vi "CRYAPI REMOVE.vi"(6 "sData":string, 8 "nData":i32, 9 "tFrame":T3, 10 "List_ID":i32[](array[numeric]), 11 "sAction":string) -> (0 "nData_Out":i32, 1 "tSpliter_Out":T1, 2 "tFrame_Out":T3, 3 "List_ID_Out":i32[](array[numeric]))   [LabVIEW 2013]
uses:
  <vilib>/Utility/miscctls.llb/LVRectTypeDef.ctl
  CRYMain Sub Window Global.vi
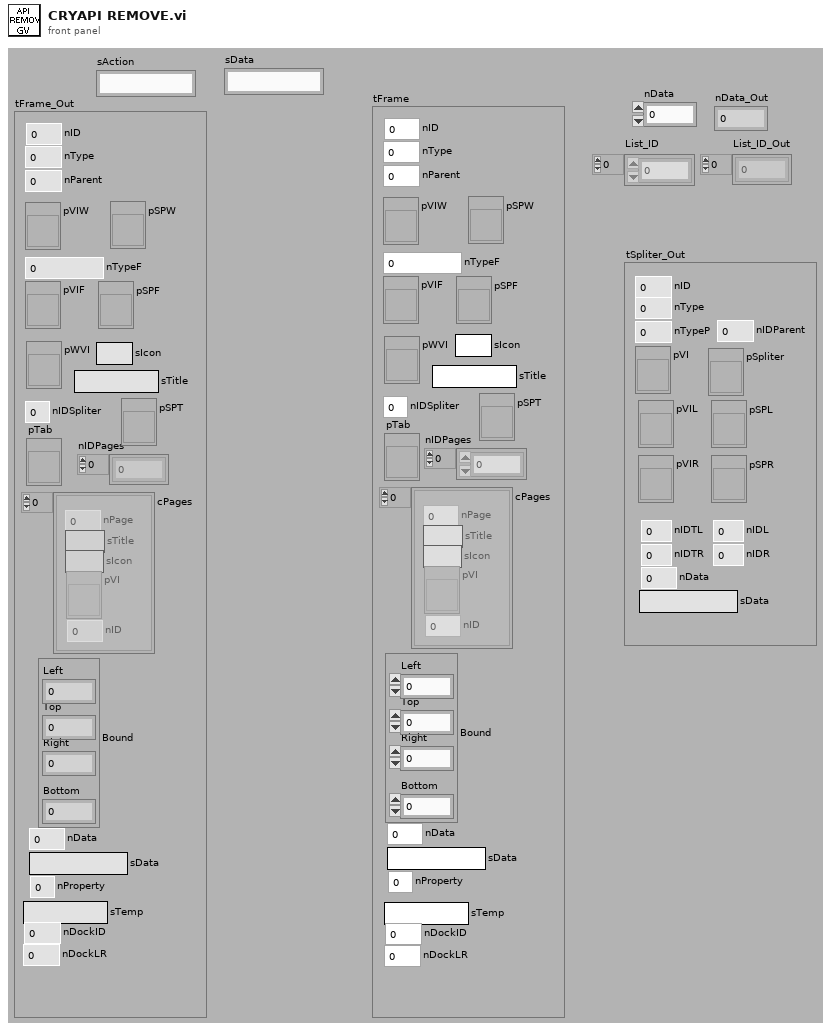
[diagram p1: front panel]
types:
  T1 = cluster{"nType":i32, "nTypeP":i32, "pVI":refnum<vi>, "pSpliter":refnum<vi>, "pSPL":refnum<vi>, "pVIL":refnum<vi>, "pSPR":refnum<vi>, "pVIR":refnum<vi>, "nIDTL":i32, "nIDL":i32, "nIDTR":i32, "nIDR":i32, "nID":i32, "nIDParent":i32, "nData":i32, "sData":string}
  T2 = typedef "LVRectTypeDef.ctl" = cluster{"Left":i16, "Top":i16, "Right":i16, "Bottom":i16}
  T3 = cluster{"nType":i32, "nParent":i32, "pVIW":refnum<vi>, "pSPW":refnum<vi>, "nTypeF":i32, "pVIF":refnum<vi>, "pSPF":refnum<vi>, "nIDSpliter":i32, "nProperty":i32, "Bound":T2, "nID":i32, "nData":i32, "sData":string, "pWVI":refnum<vi>, "sTitle":string, "cPages":cluster{"nPage":i32, "sTitle":string, "sIcon":string, "pVI":refnum<vi>, "nID":i32}[], "pTab":refnum<vi>, "nIDPages":i32[], "pSPT":refnum<vi>, "sTemp":string, "nDockID":i32, "nDockLR":i32, "sIcon":string}
  T4 = enum32{"Invalid", "Standard", "Closed", "Hidden", "Minimized", "Maximized"}
  T5 = cluster{"nPage":i32, "sTitle":string, "sIcon":string, "pVI":refnum<vi>, "nID":i32}[]
  T6 = cluster{"pSP":refnum<vi>, "pVI":refnum<vi>, "nIDT":i32, "nID":i32, "nLR":i32}
  T7 = cluster{"nID":i32[], "Frame":cluster{"nType":i32, "nParent":i32, "pVIW":refnum<vi>, "pSPW":refnum<vi>, "nTypeF":i32, "pVIF":refnum<vi>, "pSPF":refnum<vi>, "nIDSpliter":i32, "nProperty":i32, "Bound":T2, "nID":i32, "nData":i32, "sData":string, "pWVI":refnum<vi>, "sTitle":string, "cPages":cluster{"nPage":i32, "sTitle":string, "sIcon":string, "pVI":refnum<vi>, "nID":i32}[], "pTab":refnum<vi>, "nIDPages":i32[], "pSPT":refnum<vi>, "sTemp":string, "nDockID":i32, "nDockLR":i32, "sIcon":string}[]}
  T8 = cluster{"nType":i32, "nParent":i32, "pVIW":refnum<vi>, "pSPW":refnum<vi>, "nTypeF":i32, "pVIF":refnum<vi>, "pSPF":refnum<vi>, "nIDSpliter":i32, "nProperty":i32, "Bound":T2, "nID":i32, "nData":i32, "sData":string, "pWVI":refnum<vi>, "sTitle":string, "cPages":cluster{"nPage":i32, "sTitle":string, "sIcon":string, "pVI":refnum<vi>, "nID":i32}[], "pTab":refnum<vi>, "nIDPages":i32[], "pSPT":refnum<vi>, "sTemp":string, "nDockID":i32, "nDockLR":i32, "sIcon":string}[]
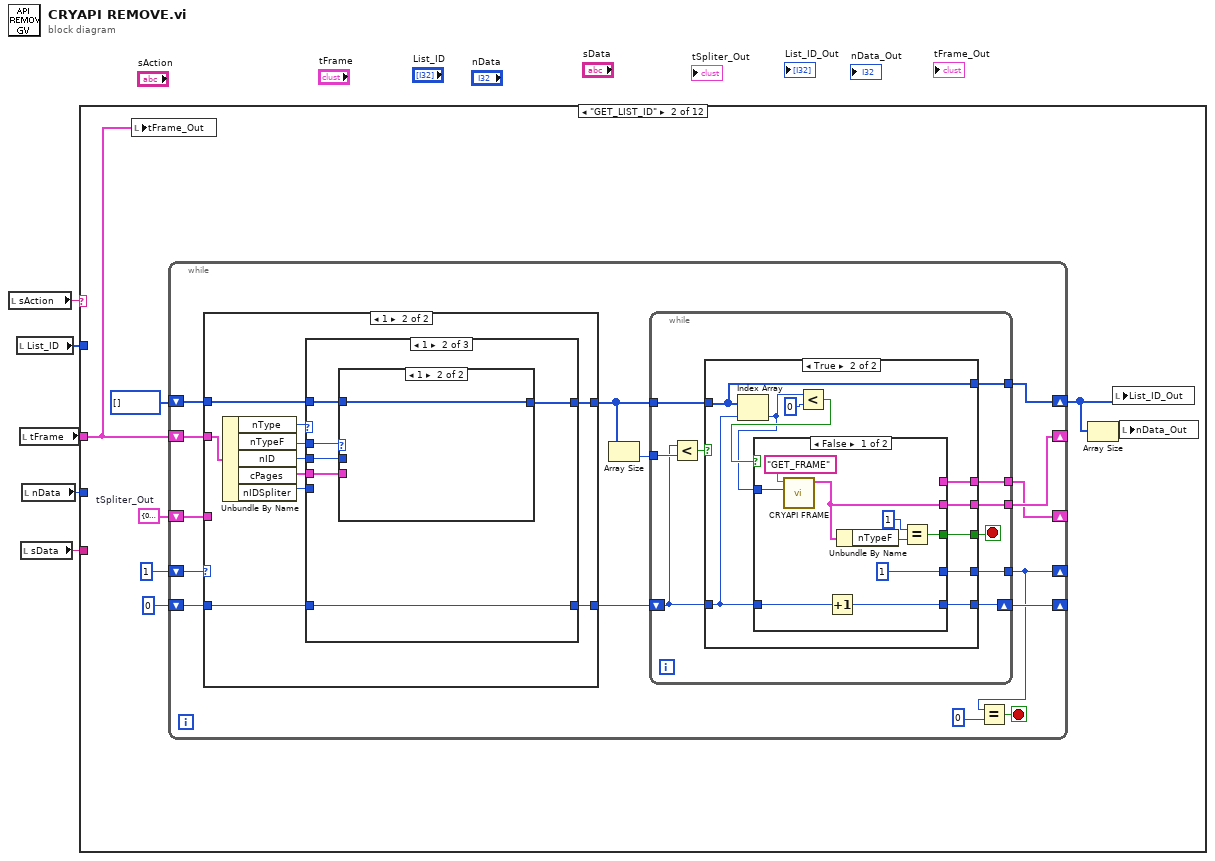
[diagram p0: block diagram]
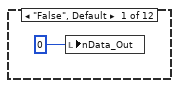
[diagram p2: hidden frame]
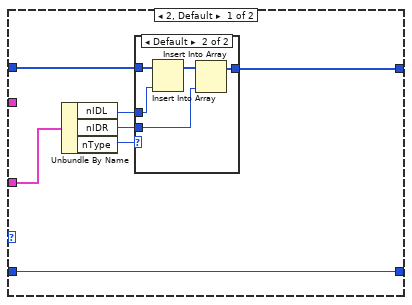
[diagram p3: hidden frame]
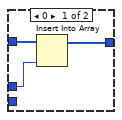
[diagram p4: hidden frame]
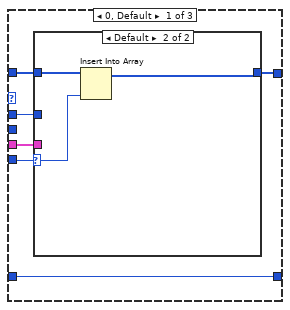
[diagram p5: hidden frame]
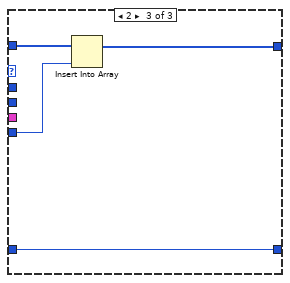
[diagram p8: hidden frame]
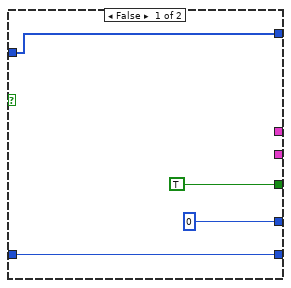
[diagram p9: hidden frame]
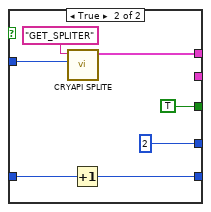
[diagram p10: hidden frame]
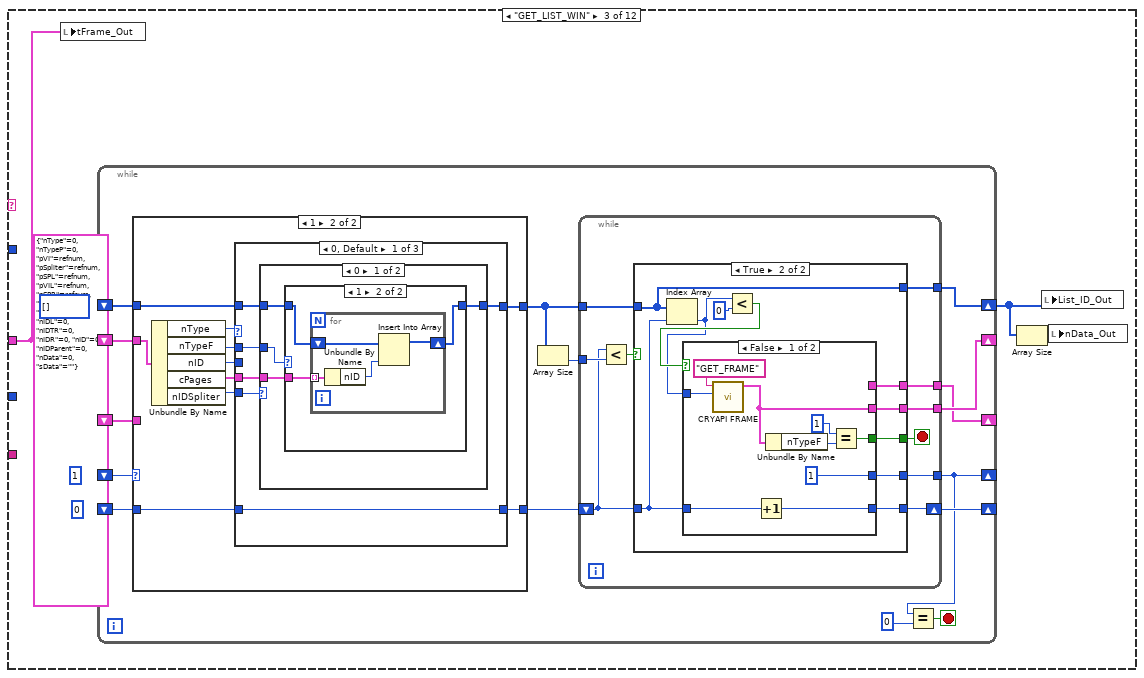
[diagram p11: hidden frame]
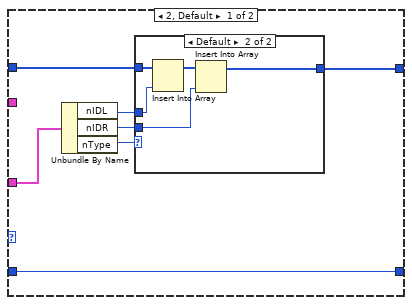
[diagram p12: hidden frame]
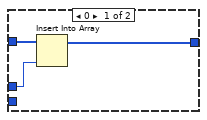
[diagram p13: hidden frame]
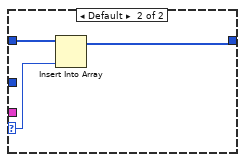
[diagram p15: hidden frame]
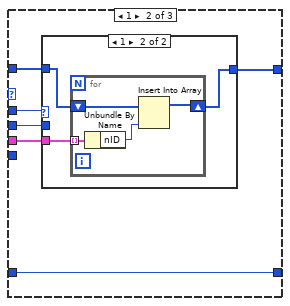
[diagram p16: hidden frame]
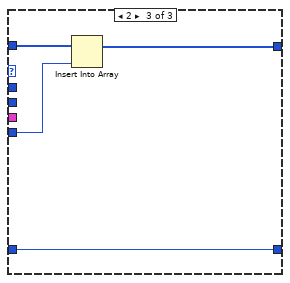
[diagram p18: hidden frame]
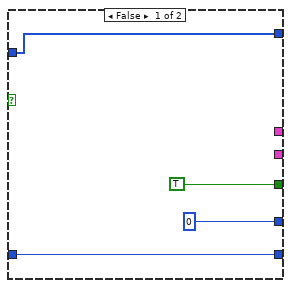
[diagram p19: hidden frame]
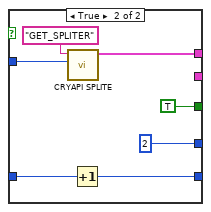
[diagram p20: hidden frame]
diagram:
  n1 = local read "sAction"() -> (w5:string)
  n2 = local read "List_ID"() -> (w3:i32[])
  n3 = local read "tFrame"() -> (w4:T3)
  n4 = local read "sData"() -> (w1:string)
  n5 = local read "nData"() -> (w2:i32)
  n6 = case shown="\"GET_LIST_ID\"" w5 {
    selector: w5 -> [_ _ _ _ w253 w299 _ _ w406 w455 w478 _]
    tunnel: w4 -> [_ w7 w116 w246 _ _ w362 _ _ _ _ _]
    tunnel: w3 -> [_ _ _ _ w255 w298 w364 w374 _ _ _ w518]
    tunnel: w2 -> [_ _ _ _ _ _ _ w379 _ _ _ w517]
    tunnel: w1 -> [_ _ _ _ _ _ _ _ _ _ _ _]
    frame "False", Default {
      n7 = local write "nData_Out"(0 ("nData_Out")) -> ()
    }
    frame "GET_LIST_ID" {
      w10 = T1 {"nType"=0, "nTypeP"=0, "pVI"=refnum, "pSpliter"=refnum, "pSPL"=refnum, "pVIL"=refnum, "pSPR"=refnum, "pVIR"=refnum, "nIDTL"=0, "nIDL"=0, "nIDTR"=0, "nIDR"=0, "nID"=0, "nIDParent"=0, "nData"=0, "sData"=""}  # tSpliter_Out
      n8 = local write "tFrame_Out"(w7) -> ()
      n9 = while {
        shift-right: [w22] -> _
        shift-left: w7 -> [w28]
        shift-right: [w14] -> w8
        shift-left: i32[] [] ("List_nID") -> [w27]
        shift-right: [w21] -> _
        shift-left: 0 -> [w26]
        shift-right: [w18] -> _
        shift-left: 1 -> [w16]
        shift-right: [w17] -> _
        shift-left: w10 -> [w15]
        stop <- w19 stop-if-true
        n10 = case shown="1" w16 {
          tunnel: w28 -> [_ w53]
          tunnel: w27 -> [w32 w49]
          tunnel: w26 -> [w30 w46]
          tunnel: [w31 w45] -> w25
          tunnel: [w30 w44] -> w23
          tunnel: w15 -> [w33 _]
          frame 2, Default {
            n11 = Unbundle By Name(w33) -> ("nIDL"=w34:i32, "nIDR"=w35:i32, "nType"=w29:i32)
            n12 = case shown="Default" w29 {
              tunnel: w35 -> [_ w43]
              tunnel: w34 -> [w38 w41]
              tunnel: w32 -> [w37 w40]
              tunnel: [w36 w39] -> w31
              frame 0 {
                n13 = Insert Into Array(array=w37, new element=w38) -> (w36:i32[])  [unwired: 1 in]
              }
              frame Default {
                n14 = Insert Into Array(array=w40, new element=w41) -> (w42:i32[])  [unwired: 1 in]
                n15 = Insert Into Array(array=w42, new element=w43) -> (w39:i32[])  [unwired: 1 in]
              }
            }
          }
          frame 1 {
            n16 = Unbundle By Name(w53) -> ("nType"=w52:i32, "nTypeF"=w51:i32, "nID"=w50:i32, "cPages"=w48:T5, "nIDSpliter"=w47:i32)
            n17 = case shown="1" w52 {
              tunnel: w51 -> [w57 w69 _]
              tunnel: w50 -> [_ w68 _]
              tunnel: w49 -> [w59 w67 w75]
              tunnel: [w56 w66 w74] -> w45
              tunnel: w48 -> [w55 w65 _]
              tunnel: w47 -> [w58 _ w72]
              tunnel: w46 -> [w54 w64 w73]
              tunnel: [w54 w64 w73] -> w44
              frame 0, Default {
                n18 = case shown="Default" w58 {
                  selector: w58 -> [_ w62]
                  tunnel: w59 -> [w60 w63]
                  tunnel: w57 -> [_ _]
                  tunnel: [w60 w61] -> w56
                  tunnel: w55 -> [_ _]
                  frame 0 {
                  }
                  frame Default {
                    n19 = Insert Into Array(array=w63, new element=w62) -> (w61:i32[])  [unwired: 1 in]
                  }
                }
              }
              frame 1 {
                n20 = case shown="1" w69 {
                  tunnel: w68 -> [_ _]
                  tunnel: w67 -> [w70 w71]
                  tunnel: [w70 w71] -> w66
                  tunnel: w65 -> [_ _]
                  frame 0, Default {
                  }
                  frame 1 {
                  }
                }
              }
              frame 2 {
                n21 = Insert Into Array(array=w75, new element=w72) -> (w74:i32[])  [unwired: 1 in]
              }
            }
          }
        }
        n22 = Array Size(array=w25) -> (size(s)=w24:i32)
        n23 = while {
          tunnel: w25 -> [w83]
          tunnel: w24 -> [w84]
          shift-right: [w78] -> w21
          shift-left: w23 -> [w82]
          tunnel: [w81] -> w17
          tunnel: [w80] -> w22
          tunnel: [w79] -> w18
          tunnel: [w76] -> w14
          stop <- w77 stop-if-true
          n24 = Less?(x=w82, y=w84) -> (x < y?=w85:bool)
          n25 = case shown="True" w85 {
            tunnel: w83 -> [w86 w90]
            tunnel: w82 -> [w88 w93]
            tunnel: [_ w96] -> w81
            tunnel: [_ w95] -> w80
            tunnel: [0 w94] -> w79
            tunnel: [w88 w92] -> w78
            tunnel: [TRUE w91] -> w77
            tunnel: [w86 w90] -> w76
            frame False {
            }
            frame True {
              n26 = Index Array(array=w90, index=w93) -> (element=w97:i32)
              n27 = Less?(x=w97, y=0) -> (x < y?=w98:bool)
              n28 = case shown="False" w98 {
                tunnel: w97 -> [w107 w114]
                tunnel: [_ w113] -> w96
                tunnel: [w103 _] -> w95
                tunnel: [1 2] -> w94
                tunnel: w93 -> [w105 w111]
                tunnel: [w104 w110] -> w92
                tunnel: [w100 TRUE] -> w91
                frame False {
                  n29 = call "CRYAPI FRAME.vi"("nData"=w107, "sAction"="GET_FRAME") -> ("tFrame_Out"=w103:T3)  [unwired: 4 in, 5 out]
                  n30 = Increment(x=w105) -> (x+1=w104:i32)
                  n31 = Unbundle By Name(w103) -> ("nTypeF"=w101:i32)
                  n32 = Equal?(x=1 ("y"), y=w101) -> (x = y?=w100:bool)
                }
                frame True {
                  n33 = call "CRYAPI SPLITE.vi"("nData"=w114, "sAction"="GET_SPLITER") -> ("tSpliter_Out"=w113:T1)  [unwired: 4 in, 5 out]
                  n34 = Increment(x=w111) -> (x+1=w110:i32)
                }
              }
            }
          }
        }
        n35 = Equal?(x=w18, y=0 ("x")) -> (x = y?=w19:bool)
      }
      n36 = Array Size(array=w8) -> (size(s)=w9:i32)
      n37 = local write "List_ID_Out"(w8) -> ()
      n38 = local write "nData_Out"(w9) -> ()
    }
    frame "GET_LIST_WIN" {
      n39 = local write "tFrame_Out"(w116) -> ()
      n40 = while {
        shift-right: [w131] -> _
        shift-left: w116 -> [w137]
        shift-right: [w123] -> w117
        shift-left: i32[] [] ("List_nID") -> [w136]
        shift-right: [w130] -> _
        shift-left: 0 -> [w135]
        shift-right: [w127] -> _
        shift-left: 1 -> [w125]
        shift-right: [w126] -> _
        shift-left: T1 {"nType"=0, "nTypeP"=0, "pVI"=refnum, "pSpliter"=refnum, "pSPL"=refnum, "pVIL"=refnum, "pSPR"=refnum, "pVIR"=refnum, "nIDTL"=0, "nIDL"=0, "nIDTR"=0, "nIDR"=0, "nID"=0, "nIDParent"=0, "nData"=0, "sData"=""} ("tSpliter_Out") -> [w124]
        stop <- w128 stop-if-true
        n41 = case shown="1" w125 {
          tunnel: w137 -> [_ w162]
          tunnel: w136 -> [w141 w158]
          tunnel: w135 -> [w139 w155]
          tunnel: [w140 w154] -> w134
          tunnel: [w139 w153] -> w132
          tunnel: w124 -> [w142 _]
          frame 2, Default {
            n42 = Unbundle By Name(w142) -> ("nIDL"=w143:i32, "nIDR"=w144:i32, "nType"=w138:i32)
            n43 = case shown="Default" w138 {
              tunnel: w144 -> [_ w152]
              tunnel: w143 -> [w147 w150]
              tunnel: w141 -> [w146 w149]
              tunnel: [w145 w148] -> w140
              frame 0 {
                n44 = Insert Into Array(array=w146, new element=w147) -> (w145:i32[])  [unwired: 1 in]
              }
              frame Default {
                n45 = Insert Into Array(array=w149, new element=w150) -> (w151:i32[])  [unwired: 1 in]
                n46 = Insert Into Array(array=w151, new element=w152) -> (w148:i32[])  [unwired: 1 in]
              }
            }
          }
          frame 1 {
            n47 = Unbundle By Name(w162) -> ("nType"=w161:i32, "nTypeF"=w160:i32, "nID"=w159:i32, "cPages"=w157:T5, "nIDSpliter"=w156:i32)
            n48 = case shown="0, Default" w161 {
              tunnel: w160 -> [w166 w189 _]
              tunnel: w159 -> [_ w188 _]
              tunnel: w158 -> [w168 w187 w201]
              tunnel: [w165 w186 w200] -> w154
              tunnel: w157 -> [w164 w185 _]
              tunnel: w156 -> [w167 _ w198]
              tunnel: w155 -> [w163 w184 w199]
              tunnel: [w163 w184 w199] -> w153
              frame 0, Default {
                n49 = case shown="0" w167 {
                  selector: w167 -> [_ w181]
                  tunnel: w168 -> [w171 w183]
                  tunnel: w166 -> [w169 _]
                  tunnel: [w170 w182] -> w165
                  tunnel: w164 -> [w172 _]
                  frame 0 {
                    n50 = case shown="1" w169 {
                      tunnel: w172 -> [_ w176]
                      tunnel: w171 -> [w173 w175]
                      tunnel: [w173 w174] -> w170
                      frame 0, Default {
                      }
                      frame 1 {
                        n51 = for {
                          tunnel: w176 -> [w180] mode=indexing
                          shift-right: [w177] -> w174
                          shift-left: w175 -> [w178]
                          n52 = Unbundle By Name(w180) -> ("nID"=w179:i32)
                          n53 = Insert Into Array(array=w178, new element=w179) -> (w177:i32[])  [unwired: 1 in]
                        }
                      }
                    }
                  }
                  frame Default {
                    n54 = Insert Into Array(array=w183, new element=w181) -> (w182:i32[])  [unwired: 1 in]
                  }
                }
              }
              frame 1 {
                n55 = case shown="1" w189 {
                  tunnel: w188 -> [_ _]
                  tunnel: w187 -> [w190 w192]
                  tunnel: [w190 w191] -> w186
                  tunnel: w185 -> [_ w193]
                  frame 0, Default {
                  }
                  frame 1 {
                    n56 = for {
                      tunnel: w193 -> [w197] mode=indexing
                      shift-right: [w194] -> w191
                      shift-left: w192 -> [w195]
                      n57 = Unbundle By Name(w197) -> ("nID"=w196:i32)
                      n58 = Insert Into Array(array=w195, new element=w196) -> (w194:i32[])  [unwired: 1 in]
                    }
                  }
                }
              }
              frame 2 {
                n59 = Insert Into Array(array=w201, new element=w198) -> (w200:i32[])  [unwired: 1 in]
              }
            }
          }
        }
        n60 = Array Size(array=w134) -> (size(s)=w133:i32)
        n61 = while {
          tunnel: w134 -> [w209]
          tunnel: w133 -> [w210]
          shift-right: [w204] -> w130
          shift-left: w132 -> [w208]
          tunnel: [w207] -> w126
          tunnel: [w206] -> w131
          tunnel: [w205] -> w127
          tunnel: [w202] -> w123
          stop <- w203 stop-if-true
          n62 = Less?(x=w208, y=w210) -> (x < y?=w211:bool)
          n63 = case shown="True" w211 {
            tunnel: w209 -> [w212 w216]
            tunnel: w208 -> [w214 w219]
            tunnel: [_ w222] -> w207
            tunnel: [_ w221] -> w206
            tunnel: [0 w220] -> w205
            tunnel: [w214 w218] -> w204
            tunnel: [TRUE w217] -> w203
            tunnel: [w212 w216] -> w202
            frame False {
            }
            frame True {
              n64 = Index Array(array=w216, index=w219) -> (element=w223:i32)
              n65 = Less?(x=w223, y=0) -> (x < y?=w224:bool)
              n66 = case shown="False" w224 {
                tunnel: w223 -> [w233 w240]
                tunnel: [_ w239] -> w222
                tunnel: [w229 _] -> w221
                tunnel: [1 2] -> w220
                tunnel: w219 -> [w231 w237]
                tunnel: [w230 w236] -> w218
                tunnel: [w226 TRUE] -> w217
                frame False {
                  n67 = call "CRYAPI FRAME.vi"("nData"=w233, "sAction"="GET_FRAME") -> ("tFrame_Out"=w229:T3)  [unwired: 4 in, 5 out]
                  n68 = Increment(x=w231) -> (x+1=w230:i32)
                  n69 = Unbundle By Name(w229) -> ("nTypeF"=w227:i32)
                  n70 = Equal?(x=1 ("y"), y=w227) -> (x = y?=w226:bool)
                }
                frame True {
                  n71 = call "CRYAPI SPLITE.vi"("nData"=w240, "sAction"="GET_SPLITER") -> ("tSpliter_Out"=w239:T1)  [unwired: 4 in, 5 out]
                  n72 = Increment(x=w237) -> (x+1=w236:i32)
                }
              }
            }
          }
        }
        n73 = Equal?(x=w127, y=0 ("x")) -> (x = y?=w128:bool)
      }
      n74 = Array Size(array=w117) -> (size(s)=w118:i32)
      n75 = local write "List_ID_Out"(w117) -> ()
      n76 = local write "nData_Out"(w118) -> ()
    }
    frame "GET_LIST_PAGES" {
      n77 = Unbundle By Name(w246) -> ("cPages"=w245:T5)
      n78 = for {
        tunnel: w245 -> [w250] mode=indexing
        shift-right: [w247] -> w242
        shift-left: i32[] [] ("List_nID") -> [w249]
        n79 = Unbundle By Name(w250) -> ("nID"=w248:i32)
        n80 = Insert Into Array(array=w249, new element=w248) -> (w247:i32[])  [unwired: 1 in]
      }
      n81 = Array Size(array=w242) -> (size(s)=w243:i32)
      n82 = local write "List_ID_Out"(w242) -> ()
      n83 = local write "nData_Out"(w243) -> ()
    }
    frame "GET_LIST_IDFRAME", "GET_LIST_IDSPLITER", "GET_LIST_IDWIN" {
      n84 = for {
        tunnel: w255 -> [w258] mode=indexing
        shift-right: [w257] -> w251
        shift-left: i32[] [] ("List_ID") -> [w260]
        tunnel: w253 -> [w256]
        n85 = case shown="\"GET_LIST_IDFRAME\"" w256 {
          tunnel: [w261 w264 w279] -> w259
          tunnel: w258 -> [w262 w265 w280]
          frame "GET_LIST_IDSPLITER", Default {
            n86 = Less?(x=w262, y=0) -> (x < y?=w261:bool)
          }
          frame "GET_LIST_IDWIN" {
            n87 = Greater?(x=w265, y=0) -> (0:w266:bool)
            n88 = case shown="True" w266 {
              tunnel: w265 -> [_ w277]
              tunnel: [FALSE w269] -> w264
              frame False {
              }
              frame True {
                n89 = call "CRYAPI FRAME.vi"("nData"=w277, "sAction"="GET_FRAME") -> ("tFrame_Out"=w276:T3)  [unwired: 4 in, 5 out]
                n90 = Unbundle By Name(w276) -> ("nType"=w274:i32, "nTypeF"=w275:i32)
                n91 = Equal?(x=1, y=w274) -> (x = y?=w270:bool)
                n92 = Equal?(x=w275, y=0 ("x")) -> (x = y?=w271:bool)
                n93 = And(x=w270, y=w271) -> (x .and. y?=w269:bool)
              }
            }
          }
          frame "GET_LIST_IDFRAME" {
            n94 = Greater?(x=w280, y=0) -> (0:w281:bool)
            n95 = case shown="True" w281 {
              tunnel: w280 -> [_ w292]
              tunnel: [FALSE w284] -> w279
              frame False {
              }
              frame True {
                n96 = call "CRYAPI FRAME.vi"("nData"=w292, "sAction"="GET_FRAME") -> ("tFrame_Out"=w291:T3)  [unwired: 4 in, 5 out]
                n97 = Unbundle By Name(w291) -> ("nType"=w289:i32, "nTypeF"=w290:i32)
                n98 = Equal?(x=2, y=w289) -> (x = y?=w285:bool)
                n99 = Equal?(x=w290, y=1 ("x")) -> (x = y?=w286:bool)
                n100 = Or(x=w285, y=w286) -> (x .or. y?=w284:bool)
              }
            }
          }
        }
        n101 = case shown="True" w259 {
          tunnel: w260 -> [w294 w297]
          tunnel: w258 -> [_ w296]
          tunnel: [w294 w295] -> w257
          frame False {
          }
          frame True {
            n102 = Insert Into Array(array=w297, new element=w296) -> (w295:i32[])  [unwired: 1 in]
          }
        }
      }
      n103 = Array Size(array=w251) -> (size(s)=w252:i32)
      n104 = local write "List_ID_Out"(w251) -> ()
      n105 = local write "nData_Out"(w252) -> ()
    }
    frame "REMOVE_FRAMES", "REMOVE_FRAME_ONLY", "REMOVE_SPF", "REMOVE_SPLITERS" {
      n106 = local write "List_ID_Out"(w298) -> ()
      n107 = for {
        tunnel: w298 -> [w301] mode=indexing
        tunnel: w299 -> [w300]
        n108 = case shown="\"REMOVE_SPF\"" w300 {
          tunnel: w301 -> [w302 w306 w311 w312]
          frame "REMOVE_FRAMES", Default {
            n109 = call "CRYAPI FRAME LIB.vi"("nData"=w302, "sAction"="REMOVE_FRAME") -> ()  [unwired: 4 in, 6 out]
          }
          frame "REMOVE_FRAME_ONLY" {
            n110 = call "CRYAPI FRAME.vi"("nData"=w306, "sAction"="GET_FRAME") -> ("tFrame_Out"=w304:T3)  [unwired: 4 in, 5 out]
            n111 = call "CRYAPI FRAME.vi"("tFrame"=w304, "sAction"="REMOVE_FRAME") -> ()  [unwired: 4 in, 6 out]
          }
          frame "REMOVE_SPLITERS" {
            n112 = call "CRYAPI SPLITE.vi"("nData"=w311, "sAction"="GET_SPLITER") -> ("tSpliter_Out"=w308:T1)  [unwired: 4 in, 5 out]
            n113 = call "CRYAPI SPLITE.vi"("tSpliter"=w308, "sAction"="REMOVE_SPLITER") -> ()  [unwired: 4 in, 6 out]
          }
          frame "REMOVE_SPF" {
            n114 = Less?(x=w312, y=0) -> (x < y?=w313:bool)
            n115 = case shown="False" w313 {
              tunnel: w312 -> [w319 w335]
              frame False {
                n116 = call "CRYAPI FRAME.vi"("nData"=w319, "sAction"="GET_FRAME") -> ("tFrame_Out"=w318:T3)  [unwired: 4 in, 5 out]
                n117 = Unbundle By Name(w318) -> ("nType"=w317:i32)
                n118 = Not Equal?(x=w317, y=1) -> (x != y?=w315:bool)
                n119 = case shown="True" w315 {
                  tunnel: w318 -> [_ w321]
                  frame False {
                  }
                  frame True {
                    n120 = Bundle By Name(cluster=w321, "nIDSpliter"=0) -> (w322:T3)
                    n121 = Unbundle By Name(w321) -> ("pSPF"=w325:refnum<vi>)
                    n122 = invoke class="SubPnl" method="Remove VI"(reference=w325) -> ()  [unwired: 2 in, 3 out]
                    n123 = call "CRYAPI FRAME.vi"("tFrame"=w322, "sAction"="REPLACE_FRAME") -> ()  [unwired: 4 in, 6 out]
                  }
                }
              }
              frame True {
                n124 = call "CRYAPI SPLITE.vi"("nData"=w335, "sAction"="GET_SPLITER") -> ("tSpliter_Out"=w326:T1)  [unwired: 4 in, 5 out]
                n125 = Unbundle By Name(w326) -> ("pSPL"=w332:refnum<vi>, "pSPR"=w331:refnum<vi>, "nType"=w333:i32, "nTypeP"=w330:i32, "nIDParent"=w328:i32)
                n126 = case shown="Default" w333 {
                  tunnel: w332 -> [w355 w359]
                  tunnel: w331 -> [_ w358]
                  tunnel: w330 -> [w354 w357]
                  tunnel: [w354 w357] -> w329
                  tunnel: w328 -> [w353 w356]
                  tunnel: [w353 w356] -> w327
                  frame 0 {
                    n127 = invoke class="SubPnl" method="Remove VI"(reference=w355) -> ()  [unwired: 2 in, 3 out]
                  }
                  frame Default {
                    n128 = invoke class="SubPnl" method="Remove VI"(reference=w358) -> ()  [unwired: 2 in, 3 out]
                    n129 = invoke class="SubPnl" method="Remove VI"(reference=w359) -> ()  [unwired: 2 in, 3 out]
                  }
                }
                n130 = case shown="0, Default" w329 {
                  tunnel: w327 -> [w341 w350]
                  tunnel: w326 -> [_ w348]
                  frame 0, Default {
                    n131 = call "CRYAPI FRAME.vi"("nData"=w341, "sAction"="GET_FRAME") -> ("tFrame_Out"=w337:T3)  [unwired: 4 in, 5 out]
                    n132 = Unbundle By Name(w337) -> ("pSPF"=w336:refnum<vi>)
                    n133 = invoke class="SubPnl" method="Remove VI"(reference=w336) -> ()  [unwired: 2 in, 3 out]
                    n134 = Bundle By Name(cluster=w337, "nParent"=0 ("nIDSpliter")) -> (w338:T3)
                    n135 = call "CRYAPI FRAME.vi"("tFrame"=w338, "sAction"="REPLACE_FRAME") -> ()  [unwired: 4 in, 6 out]
                  }
                  frame 1 {
                    n136 = call "CRYAPI SPLITE.vi"("nData"=w350, "sAction"="GET_SPLITER") -> ("tSpliter_Out"=w347:T1)  [unwired: 4 in, 5 out]
                    n137 = call "CRYAPI SPLITE.vi"("tSpliter_In"=w348, "tSpliter"=w347, "sAction"="GET_SPLITER_LR") -> ("tLR_Out"=w346:T6)  [unwired: 3 in, 5 out]
                    n138 = Unbundle By Name(w346) -> ("pSP"=w345:refnum<vi>, "nIDT"=w344:i32)
                    n139 = Greater Than 0?(x=w344) -> (x > 0?=w343:bool)
                    n140 = case shown="True" w343 {
                      tunnel: w345 -> [_ w352]
                      frame False {
                      }
                      frame True {
                        n141 = invoke class="SubPnl" method="Remove VI"(reference=w352) -> ()  [unwired: 2 in, 3 out]
                      }
                    }
                  }
                }
              }
            }
          }
        }
      }
    }
    frame "INSERT_PAGES" {
      n142 = local write "nData_Out"(1 ("nData_Out")) -> ()
      n143 = local write "List_ID_Out"(w364) -> ()
      n144 = for {
        tunnel: w364 -> [w372] mode=indexing
        shift-right: [w365] -> w360
        shift-left: w362 -> [w366]
        n145 = call "CRYAPI FRAME.vi"("nData"=w372, "sAction"="GET_FRAME") -> ("tFrame_Out"=w370:T3)  [unwired: 4 in, 5 out]
        n146 = Bundle By Name(cluster=w370, "nParent"=0) -> (w367:T3)
        n147 = call "CRYAPI FRAME LIB.vi"("tFrame_In"=w367, "tFrame"=w366, "sAction"="INSERT_PAGE") -> ("tFrame_Out"=w365:T3)  [unwired: 3 in, 5 out]
        n148 = call "CRYAPI FRAME.vi"("tFrame"=w367, "sAction"="REPLACE_FRAME") -> ()  [unwired: 4 in, 6 out]
      }
      n149 = local write "tFrame_Out"(w360) -> ()
      n150 = call "CRYAPI FRAME.vi"("tFrame"=w360, "sAction"="REPLACE_FRAME") -> ()  [unwired: 4 in, 6 out]
    }
    frame "FIND_SPLITER" {
      n151 = local write "List_ID_Out"(w374) -> ()
      n152 = for {
        tunnel: w374 -> [w387] mode=indexing
        tunnel: w379 -> [w386]
        tunnel: [w385] -> w378
        tunnel: [w383] -> w376
        tunnel: [w382] -> w377
        i -> [w384]
        stop <- w382 stop-if-true
        n153 = Less?(x=w387, y=0) -> (x < y?=w388:bool)
        n154 = case shown="True" w388 {
          tunnel: w387 -> [_ w401]
          tunnel: w386 -> [_ w398]
          tunnel: [FALSE w395] -> w382
          tunnel: [T1 {"nType"=0, "nTypeP"=0, "pVI"=refnum, "pSpliter"=refnum, "pSPL"=refnum, "pVIL"=refnum, "pSPR"=refnum, "pVIR"=refnum, "nIDTL"=0, "nIDL"=0, "nIDTR"=0, "nIDR"=0, "nID"=0, "nIDParent"=0, "nData"=0, "sData"=""} ("tSpliter_Out") w394] -> w385
          tunnel: w384 -> [_ w393]
          tunnel: [0 w393] -> w383
          frame False {
          }
          frame True {
            n155 = call "CRYAPI SPLITE.vi"("nData"=w401, "sAction"="GET_SPLITER") -> ("tSpliter_Out"=w394:T1)  [unwired: 4 in, 5 out]
            n156 = Unbundle By Name(w394) -> ("nIDL"=w400:i32, "nIDR"=w399:i32)
            n157 = Equal?(x=w400, y=w398) -> (x = y?=w397:bool)
            n158 = Equal?(x=w399, y=w398) -> (x = y?=w396:bool)
            n159 = Or(x=w397, y=w396) -> (x .or. y?=w395:bool)
          }
        }
      }
      n160 = local write "tSpliter_Out"(w378) -> ()
      n161 = case shown="False" w377 {
        tunnel: w376 -> [_ w381]
        tunnel: [-1 w381] -> w375
        frame False {
        }
        frame True {
        }
      }
      n162 = local write "nData_Out"(w375) -> ()
    }
    frame "MAXIMIZE_FRAMES", "MINIMIZE_FRAMES" {
      n163 = global read "CRYMain Sub Window Global.vi" "cFrame"() -> (w405:T7)
      n164 = Unbundle By Name(w405) -> ("Frame"=w404:T8)
      n165 = for {
        tunnel: w404 -> [w426] mode=indexing
        tunnel: w406 -> [w427]
        tunnel: [w421] -> w403
        n166 = Unbundle By Name(w426) -> ("nType"=w425:i32, "nParent"=w429:i32, "pVIW"=w428:refnum<vi>)  [unwired: 1 out]
        n167 = Not Equal To 0?(x=w425) -> (x != 0?=w424:bool)
        n168 = Equal To 0?(x=w429) -> (x = 0?=w423:bool)
        n169 = And(x=w424, y=w423) -> (x .and. y?=w422:bool)
        n170 = case shown="True" w422 {
          tunnel: w428 -> [_ w433]
          tunnel: w427 -> [w430 w431]
          tunnel: w426 -> [_ w432]
          tunnel: [w430 w431] -> w421
          frame False {
          }
          frame True {
            n171 = case shown="\"MAXIMIZE_FRAMES\"" w431 {
              tunnel: w433 -> [_ w438 w443]
              tunnel: w432 -> [_ w437 w441]
              frame "False", Default {
              }
              frame "MAXIMIZE_FRAMES" {
                n172 = Unbundle By Name(w437) -> ("sData"=w436:string)
                n173 = Equal?(x=w436, y="Minimized" ("sData")) -> (x = y?=w434:bool)
                n174 = case shown="True" w434 {
                  tunnel: w438 -> [_ w440]
                  frame False {
                  }
                  frame True {
                    n175 = property class="VI"(reference=w440, "FP.State"=T4."Standard" ("Front Panel Window:State")) -> ()  [unwired: 1 in, 2 out]
                  }
                }
              }
              frame "MINIMIZE_FRAMES" {
                n176 = property class="VI"(reference=w443) -> ("FP.State"=w445:T4)  [unwired: 1 in, 2 out]
                n177 = Equal?(x=w445, y=T4."Standard" ("Front Panel Window:State")) -> (x = y?=w442:bool)
                n178 = case shown="True" w442 {
                  tunnel: w443 -> [_ w450]
                  tunnel: w441 -> [_ w449]
                  frame False {
                  }
                  frame True {
                    n179 = Bundle By Name(cluster=w449, "sData"="Minimized") -> (w446:T3)
                    n180 = property class="VI"(reference=w450, "FP.State"=T4."Hidden" ("Front Panel Window:State")) -> ()  [unwired: 1 in, 2 out]
                    n181 = call "CRYAPI FRAME.vi"("tFrame"=w446, "sAction"="REPLACE_FRAME") -> ()  [unwired: 4 in, 6 out]
                  }
                }
              }
            }
          }
        }
      }
      n182 = case shown="\"MAXIMIZE_FRAMES\"" w403 {
        frame "False", Default {
        }
        frame "MAXIMIZE_FRAMES" {
          n183 = global read "CRYMain Sub Window Global.vi" "ActiveWID"() -> (w407:i32)
          n184 = Greater Than 0?(x=w407) -> (x > 0?=w408:bool)
          n185 = case shown="True" w408 {
            tunnel: w407 -> [_ w409]
            frame False {
            }
            frame True {
              n186 = call "CRYAPI FRAME.vi"("nData"=w409, "sAction"="GET_FRAME") -> ("tFrame_Out"=w417:T3)  [unwired: 4 in, 5 out]
              n187 = Unbundle By Name(w417) -> ("pVIW"=w416:refnum<vi>, "nParent"=w413:i32)
              n188 = property class="VI"(reference=w416) -> ("FP.State"=w414:T4)  [unwired: 1 in, 2 out]
              n189 = Equal?(x=w414, y=T4."Standard" ("Front Panel Window:State")) -> (x = y?=w410:bool)
              n190 = Not Equal To 0?(x=w413) -> (x != 0?=w411:bool)
              n191 = Or(x=w411, y=w410) -> (x .or. y?=w412:bool)
              n192 = case shown="True" w412 {
                tunnel: w409 -> [_ w419]
                frame False {
                }
                frame True {
                  n193 = call "CRYAPI FRAME LIB.vi"("nData"=w419, "sAction"="ACTIVE_FRAME_ID") -> ()  [unwired: 4 in, 6 out]
                }
              }
            }
          }
        }
      }
    }
    frame "GET_FLOAT_FRAMES" {
      n194 = global read "CRYMain Sub Window Global.vi" "cFrame"() -> (w457:T7)
      n195 = Unbundle By Name(w457) -> ("Frame"=w456:T8)
      n196 = for {
        tunnel: w456 -> [w466] mode=indexing
        tunnel: w455 -> [w467]
        tunnel: [w464] -> _
        shift-right: [w461] -> w453
        shift-left: i32[] [] ("List_ID_Out") -> [w463]
        n197 = Unbundle By Name(w466) -> ("nID"=w462:i32, "nType"=w465:i32, "nParent"=w468:i32)
        n198 = Not Equal To 0?(x=w465) -> (x != 0?=w459:bool)
        n199 = Equal To 0?(x=w468) -> (x = 0?=w460:bool)
        n200 = Compound Arithmetic op=AND(w459, w460) -> (w458:bool)
        n201 = case shown="True" w458 {
          tunnel: w467 -> [w470 w474]
          tunnel: [w470 w474] -> w464
          tunnel: w463 -> [w469 w473]
          tunnel: w462 -> [_ w472]
          tunnel: [w469 w471] -> w461
          frame False {
          }
          frame True {
            n202 = Insert Into Array(array=w473, new element=w472) -> (w471:i32[])  [unwired: 1 in]
          }
        }
      }
      n203 = Array Size(array=w453) -> (size(s)=w452:i32)
      n204 = local write "List_ID_Out"(w453) -> ()
      n205 = local write "nData_Out"(w452) -> ()
    }
    frame "GET_FRAME_FRAMES", "GET_TAB_FRAMES", "GET_WIN_FRAMES" {
      n206 = global read "CRYMain Sub Window Global.vi" "cFrame"() -> (w480:T7)
      n207 = Unbundle By Name(w480) -> ("Frame"=w479:T8)
      n208 = for {
        tunnel: w479 -> [w486] mode=indexing
        tunnel: w478 -> [w481]
        shift-right: [w483] -> w476
        shift-left: i32[] [] ("List_ID_Out") -> [w485]
        n209 = case shown="\"GET_FRAME_FRAMES\"" w481 {
          tunnel: w486 -> [_ w497 w502 w510]
          tunnel: [0 ("nID") w496 w501 w509] -> w484
          tunnel: [FALSE w489 w498 w506] -> w482
          frame "False", Default {
          }
          frame "GET_WIN_FRAMES" {
            n210 = Unbundle By Name(w497) -> ("nID"=w496:i32, "nType"=w495:i32, "nTypeF"=w493:i32)
            n211 = Equal?(x=w495, y=1) -> (x = y?=w490:bool)
            n212 = Equal?(x=w493, y=0) -> (x = y?=w491:bool)
            n213 = And(x=w490, y=w491) -> (x .and. y?=w489:bool)
          }
          frame "GET_TAB_FRAMES" {
            n214 = Unbundle By Name(w502) -> ("nID"=w501:i32, "nTypeF"=w500:i32)
            n215 = Equal?(x=w500, y=1) -> (x = y?=w498:bool)
          }
          frame "GET_FRAME_FRAMES" {
            n216 = Unbundle By Name(w510) -> ("nID"=w509:i32, "nTypeF"=w508:i32, "nType"=w504:i32)
            n217 = case shown="Default" w504 {
              tunnel: [TRUE FALSE] -> w503
              frame 0, 2 {
              }
              frame Default {
              }
            }
            n218 = Not Equal?(x=w508, y=1) -> (x != y?=w505:bool)
            n219 = And(x=w505, y=w503) -> (x .and. y?=w506:bool)
          }
        }
        n220 = case shown="True" w482 {
          tunnel: w485 -> [w513 w516]
          tunnel: w484 -> [_ w515]
          tunnel: [w513 w514] -> w483
          frame False {
          }
          frame True {
            n221 = Insert Into Array(array=w516, new element=w515) -> (w514:i32[])  [unwired: 1 in]
          }
        }
      }
      n222 = Array Size(array=w476) -> (size(s)=w475:i32)
      n223 = local write "List_ID_Out"(w476) -> ()
      n224 = local write "nData_Out"(w475) -> ()
    }
    frame "SET_ACTIVENUMBERS" {
      n225 = for {
        tunnel: w518 -> [w519] mode=indexing
        tunnel: w517 -> [w521]
        n226 = Greater Than 0?(x=w519) -> (x > 0?=w520:bool)
        n227 = case shown="True" w520 {
          tunnel: w519 -> [_ w527]
          tunnel: w521 -> [_ w524]
          frame False {
          }
          frame True {
            n228 = call "CRYAPI FRAME.vi"("nData"=w527, "sAction"="GET_FRAME") -> ("tFrame_Out"=w526:T3)  [unwired: 4 in, 5 out]
            n229 = Unbundle By Name(w526) -> ("pVIW"=w525:refnum<vi>, "nType"=w522:i32)  [unwired: 1 out]
            n230 = Greater Than 0?(x=w522) -> (x > 0?=w523:bool)
            n231 = case shown="True" w523 {
              tunnel: w525 -> [_ w530]
              tunnel: w524 -> [_ w529]
              frame False {
              }
              frame True {
                n232 = invoke class="VI" method="Ctrl Val.Set"(reference=w530, "Control Name"="ActiveNumber", "Value"=w529) -> ()  [unwired: 2 in, 5 out]
              }
            }
          }
        }
      }
    }
  }
